vi "G# - GarbageCollectorDemo.vi"() -> ()   [LabVIEW 2017]
doc: "Garbage Collector\nThis examples shows how the garbage collector could be used to destroy all objects.\n\nThis implementation is more a \"Java\" or \"C#\" stylish way of programming, where the destruction of created objects is of less concern.\n\nThe indicator \"# of objects killed\" will show the difference in execution.\n\nBy using the G# Debugger found in Tools->G# Debugger a text log can be followed showing how the objects were created and destroyed. This is a good way of understanding the difference between garbage collection and a implemented destroy function for all objects."
uses:
  <vilib>/addons/_AddQ/G#Object/G#Object.lvclass
  MyG#G3SubTempl_class/MyG#G3SubTempl.lvclass
  C:/Program Files/National Instruments/LabVIEW 2017/vi.lib/addons/_AddQ/G#Object/G#Object.lvclass
  MyG#G3Templ_class/MyG#G3Templ.lvclass
  MyG#Class_class/MyG#Class.lvclass
  MyG#SubClass_class/MyG#SubClass.lvclass
panel:
  in  "error in (no error)":errorcluster
  out "error out":errorcluster
  out "OK":bool
  out "# of objects killed":i32
  in  "Let garbage collector do all work?":bool=TRUE
  # "Garbage Collector\nThis examples shows how the garbage collector could be used to destroy all objects.\n\nThis implementation is more a  \"Java\" or \"C#\" stylish way of programming, where the destruction of created objects is of less concern.\n\nThe indicator \"# of objects killed\" will show the difference in execution.\n\nBy using the G# Debugger found in Tools->G# Debugger a text log can be followed showing how the objects were created and destroyed.\nThis is a good way of understanding the difference between garbage collection and a implemented destroy function for all objects."
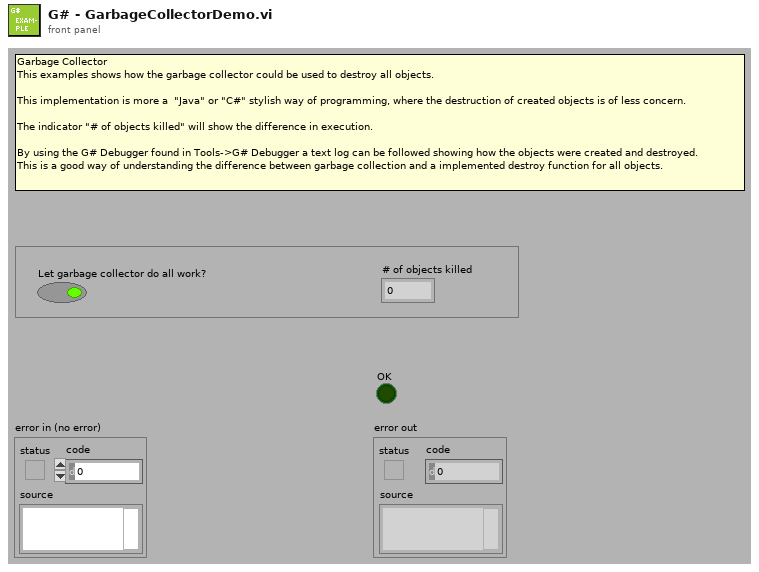
[diagram p1: front panel]
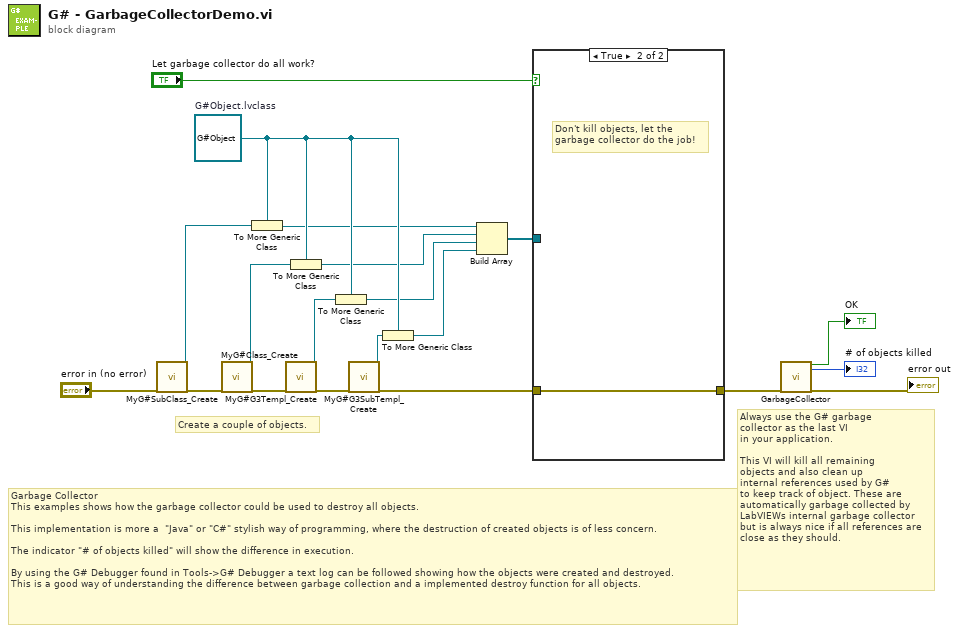
[diagram p0: block diagram]
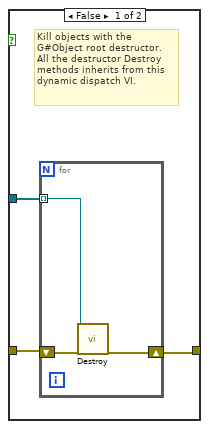
[diagram p2: hidden frame]
diagram:
  w15 = refnum<class "G#Object.lvclass"> refnum  # G#Object.lvclass
  # "Garbage Collector\nThis examples shows how the garbage collector could be used to destroy all objects.\n\nThis implementation is more a  \"Java\" or \"C#\" stylish way of programming, where the destruction of created objects is of less concern.\n\nThe indicator \"# of objects killed\" will show the difference in execution.\n\nBy using the G# Debugger found in Tools->G# Debugger a text log can be followed showing how the objects were created and destroyed.\nThis is a good way of understanding the difference between garbage collection and a implemented destroy function for all objects."
  # "Create a couple of objects."
  # "Always use the G# garbage\ncollector as the last VI\nin your application.\n\nThis VI will kill all remaining\nobjects and also clean up\ninternal references used by G#\nto keep track of object. These are\nautomatically garbage collected by\nLabVIEWs internal garbage collector\nbut is always nice if all references are\nclose as they should."
  n1 = call "MyG#SubClass_Create.vi"("error in (no error)"="error in (no error)") -> ("reference out"=w17:refnum<class "MyG#SubClass.lvclass">, "error out"=w20:errorcluster)  [unwired: 17 in]
  n2 = call "MyG#Class_Create.vi"("error in (no error)"=w20) -> ("reference out"=w16:refnum<class "MyG#Class.lvclass">, "error out"=w19:errorcluster)  [unwired: 17 in]
  n3 = To More Generic Class(target class=w15, reference=w17) -> (generic class reference=w12:refnum<class "G#Object.lvclass">)
  n4 = call "MyG#G3Templ_Create.vi"("error in (no error)"=w19) -> ("reference out"=w14:refnum<class "MyG#G3Templ.lvclass">, "error out"=w18:errorcluster)  [unwired: 17 in]
  n5 = To More Generic Class(target class=w15, reference=w16) -> (generic class reference=w11:refnum<class "G#Object.lvclass">)
  n6 = To More Generic Class(target class=w15, reference=w14) -> (generic class reference=w10:refnum<class "G#Object.lvclass">)
  n7 = call "MyG#G3SubTempl_Create.vi"("error in (no error)"=w18) -> ("reference out"=w13:refnum<class "MyG#G3SubTempl.lvclass">, "error out"=w8:errorcluster)  [unwired: 17 in]
  n8 = To More Generic Class(target class=w15, reference=w13) -> (generic class reference=w9:refnum<class "G#Object.lvclass">)
  n9 = Build Array(w12, w11, w10, w9) -> (w5:refnum<class "G#Object.lvclass">[])
  n10 = case shown="True" "Let garbage collector do all work?" {
    tunnel: w8 -> [w23 w27]
    tunnel: [w21 w27] -> w7
    tunnel: w5 -> [w22 _]
    frame False {
      # "Kill objects with the\nG#Object root destructor.\nAll the destructor Destroy\nmethods inherits from this\ndynamic dispatch VI."
      n11 = for {
        shift-right: [w25] -> w21
        shift-left: w23 -> [w26]
        tunnel: w22 -> [w24] mode=indexing
        n12 = call-dynamic "Destroy.vi"("reference in"=w24, "error in (no error)"=w26) -> ("error out"=w25:errorcluster)  [unwired: 16 in, 1 out]
      }
    }
    frame True {
      # "Don't kill objects, let the\ngarbage collector do the job!"
    }
  }
  n13 = call <vilib>:"GarbageCollector.vi"("error in (no error)"=w7) -> ("OK"=→"OK":bool, "# of objects killed"=→"# of objects killed":i32, "error out"=→"error out":errorcluster)  [unwired: 16 in]
